vi "Example SM.vi"() -> ()   [LabVIEW 2020]
uses:
  FINS/FINS_header.ctl
  FINS/FINS CMD.ctl
  subvi/task.ctl
  FINS/FINS TCP.lvlib
panel:
  out "Waveform Chart 2":u32(graph)
  out "x-y 2":u32
  out "Array":sgl[](array[numeric])
  out "x-y":u32
  in  "address":u16=146
  out "Waveform Chart":sgl[][](graph)
  in  "stop":bool
  out "error o":errorcluster
  out "Numeric":sgl format="%.1f"
  out "data":bool[][](array[boolean])
  out "data":u8[](array[numeric])
  out "RSP":bool
  out "server Header":T1={"resp req"=FALSE, "cmd resp"=FALSE, "SID"=255, "DNA"=2, "DA1"=2, "DA2"=2, "SA1"=0, "SA2"=255, "SNA"=255} {"SNA" max=127 format="%x"; "SA2" max=254 step=1 format="%x"; "SA1" format="%x"; "DA2" max=254 step=1 format="%x"; "DA1" format="%x"; "DNA" max=127 step=1 format="%x"}
  out "server CMD":T2
  out "FINS Header":T1 {"SNA" max=127 format="%x"; "SA2" max=254 step=1 format="%x"; "SA1" format="%x"; "DA2" max=254 step=1 format="%x"; "DA1" format="%x"; "DNA" max=127 step=1 format="%x"}
  in  "SA1":u8 format="%x"
  out "Client Node":u32=10 format="%x"
  out "Server Node":u32=10 format="%x"
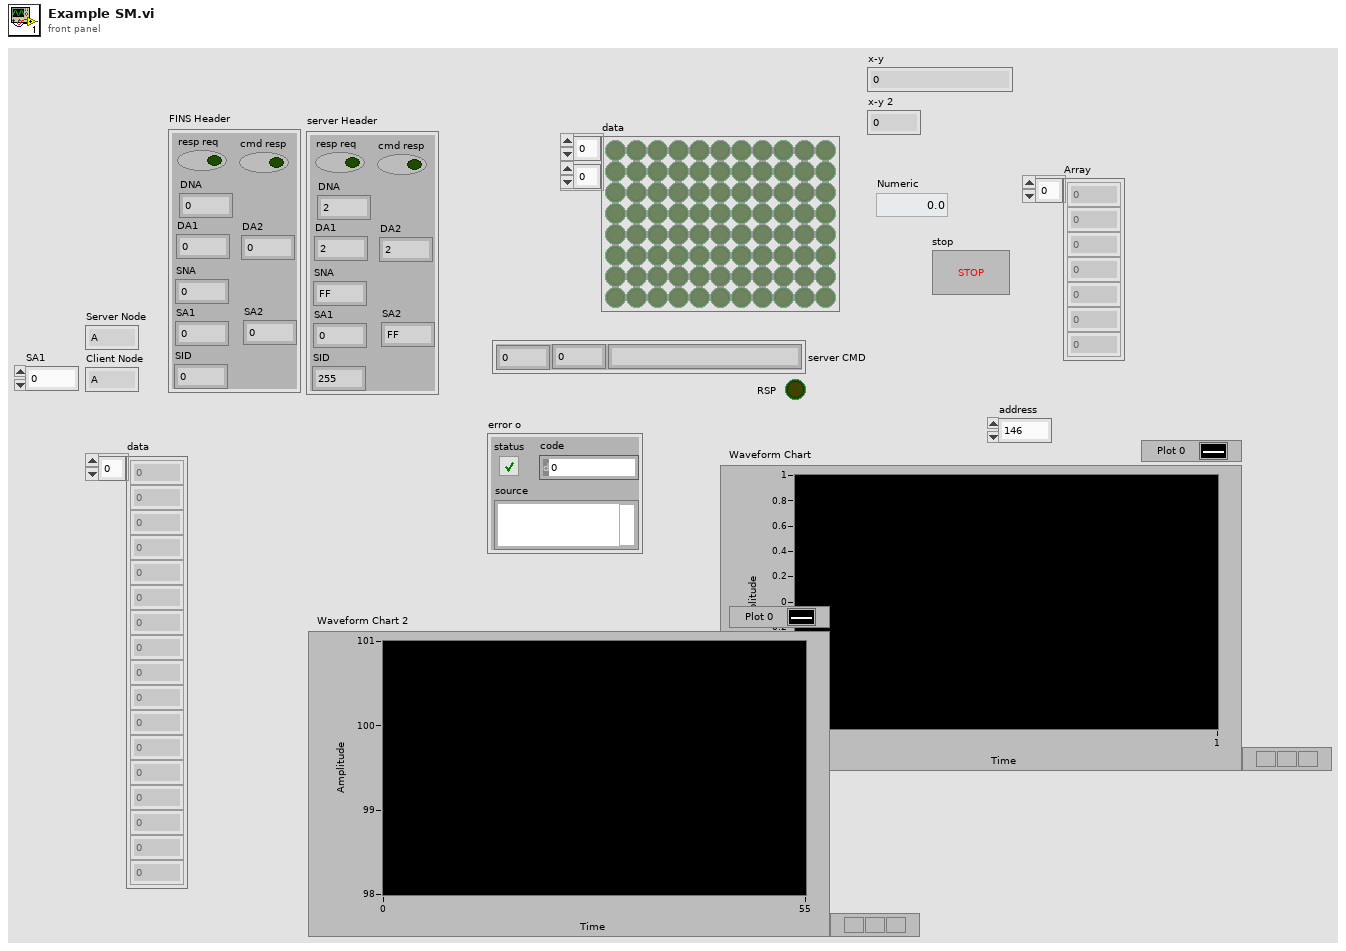
[diagram p1: front panel]
types:
  T1 = typedef "FINS TCP.lvlib/FINS_header.ctl" = cluster{"resp req":bool, "cmd resp":bool, "SID":u8, "DNA":u8, "DA1":u8, "DA2":u8, "SA1":u8, "SA2":u8, "SNA":u8}
  T2 = typedef "FINS TCP.lvlib/FINS CMD.ctl" = cluster{"MR":u8, "SR":u8, "name":string}
  T3 = typedef "task.ctl" = enum16{"connect", "send", "send-recv", "receive", "disconnect"}
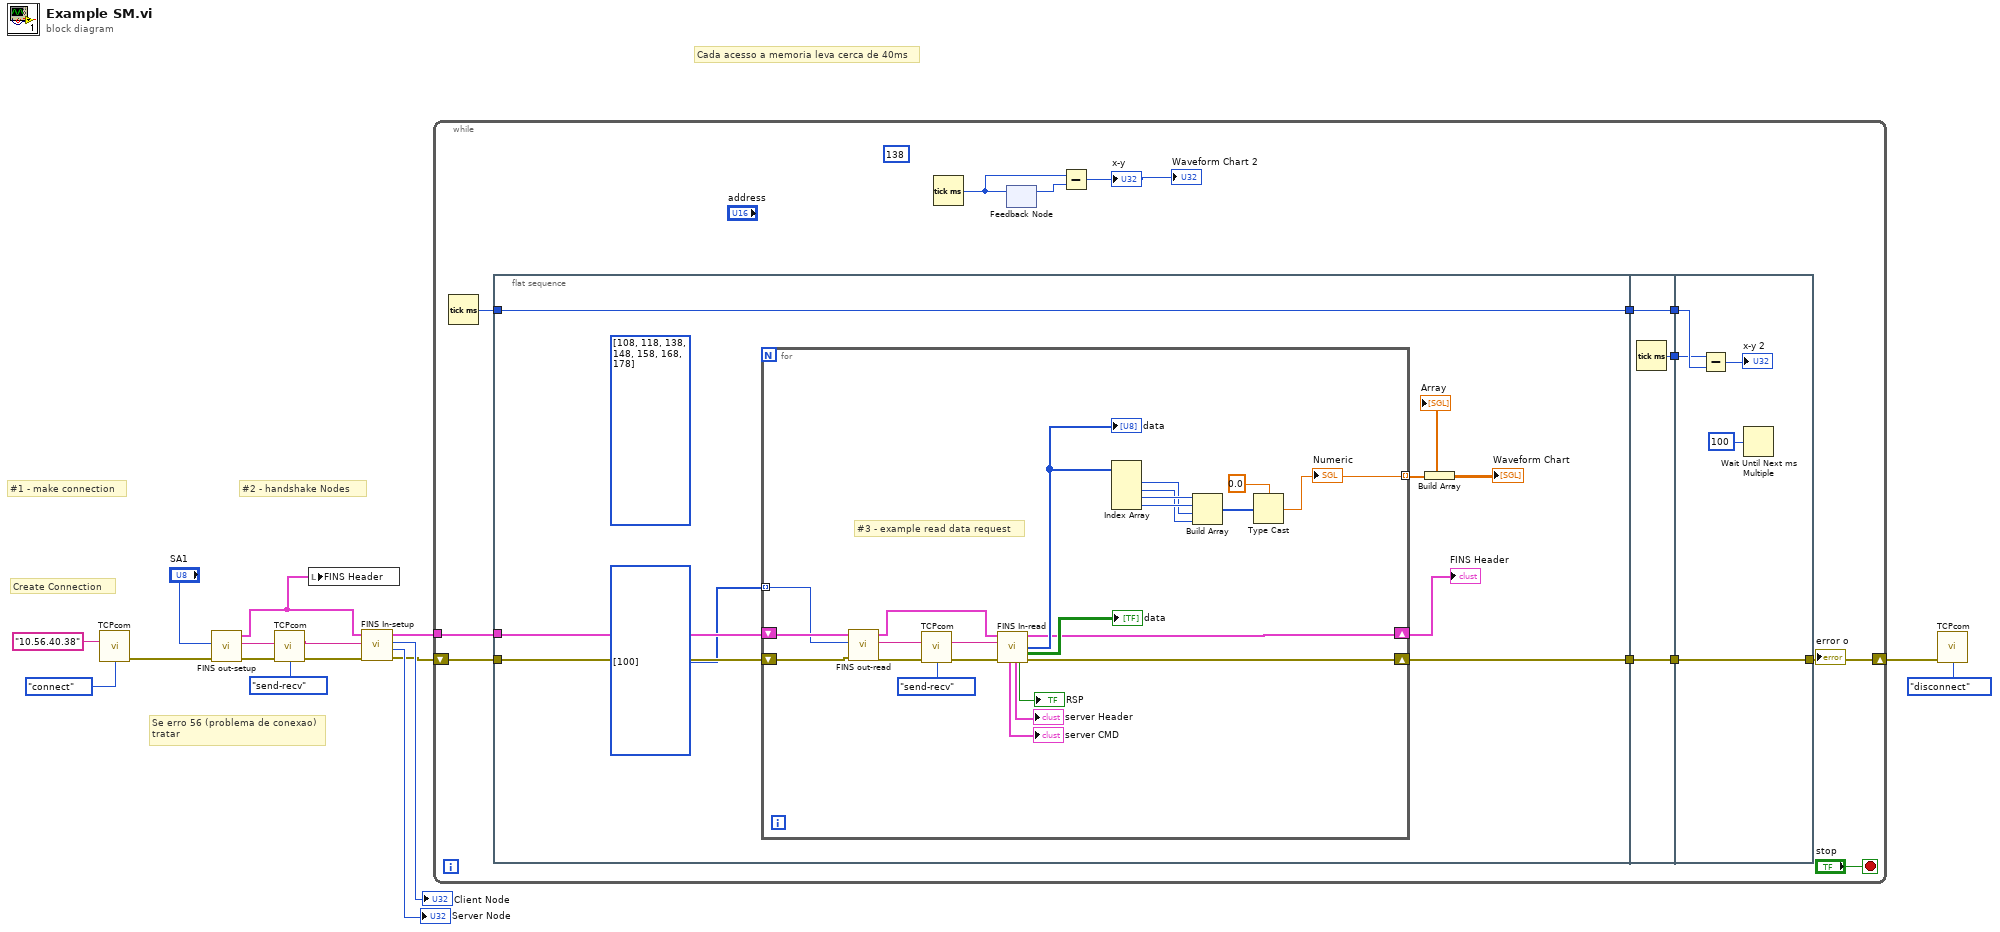
[diagram p0: block diagram]
diagram:
  # "Cada acesso a memoria leva cerca de 40ms"
  # "Se erro 56 (problema de conexao)\ntratar"
  # "#2 - handshake Nodes"
  # "#1 - make connection"
  # "Create Connection"
  n1 = call "TCPcom.vi"("string"="10.56.40.38" ("address"), "task"=task."connect") -> ("error out"=w15:errorcluster)  [unwired: 12 in, 1 out]
  n2 = call "FINS out-setup.vi"("error i"=w15, "SA1"="SA1") -> ("error o"=w13:errorcluster, "msg"=w14:string, "FINS Header"=w3:T1)  [unwired: 7 in]
  n3 = call "TCPcom.vi"("string"=w14, "error in"=w13, "task"=task."send-recv") -> ("data out"=w11:string, "error out"=w10:errorcluster)  [unwired: 11 in]
  n4 = local write "FINS Header"(w3) -> ()
  n5 = call "FINS In-setup.vi"("error i"=w10, "msg 3"=w11, "FINS Header i"=w3) -> ("error o"=w4:errorcluster, "Server Node"=→"Server Node":u32, "Client Node"=→"Client Node":u32, "FINS Header o"=w5:T1)  [unwired: 5 in]
  n6 = while {
    tunnel: w5 -> [w29]
    shift-right: [w27] -> w1
    shift-left: w4 -> [w28]
    stop <- "stop" stop-if-true
    (unwired) u16 138 ("address")
    n7 = Tick Count (ms)() -> (millisecond timer value=w23:u32)
    n8 = flat-sequence {
      tunnel: w29 -> [w37]
      tunnel: w28 -> [w36]
      tunnel: [w35] -> w22
      tunnel: [w30] -> w20
      tunnel: w23 -> [w30]
      tunnel: w22 -> [w63]
      tunnel: [w63] -> w21
      tunnel: w20 -> [w62]
      tunnel: [w62] -> w19
      tunnel: [w61] -> w18
      tunnel: [w68] -> w27
      tunnel: w21 -> [w68]
      tunnel: w19 -> [w66]
      tunnel: w18 -> [w65]
      frame #0 {
        (unwired) u16[] [108, 118, 138, 148, 158, 168, 178]
        n9 = for {
          shift-right: [w50] -> w35
          shift-left: w36 -> [w58]
          tunnel: u16[] [100] -> [w40] mode=indexing
          tunnel: [w39] -> w33 mode=indexing
          shift-right: [w38] -> w31
          shift-left: w37 -> [w59]
          # "#3 - example read data request"
          n10 = call "FINS out-read.vi"("error i"=w58, "address"=w40, "FINS Header 2"=w59) -> ("error o"=w56:errorcluster, "msg"=w57:string, "FINS Header"=w49:T1)  [unwired: 6 in]
          n11 = call "TCPcom.vi"("string"=w57, "error in"=w56, "task"=task."send-recv") -> ("data out"=w55:string, "error out"=w54:errorcluster)  [unwired: 11 in]
          n12 = call "FINS In-read.vi"("FINS Header i"=w49, "msg 3"=w55, "error i"=w54) -> ("FINS Header o"=w38:T1, 8:"data"=w41:u8[], 10:"data"=→"data":bool[][], "CMD"=→"server CMD":T2, "FINS Header 2"=→"server Header":T1, "RSP"=→"RSP":bool, "error o"=w50:errorcluster)  [unwired: 6 in]
          "data" <- w41
          n13 = Index Array(array=w41) -> (element #1=w44:u8, element #2=w43:u8, element #3=w46:u8, element #4=w45:u8)  [unwired: 4 in]
          n14 = Build Array(w46, w45, w44, w43) -> (w42:u8[])
          n15 = Type Cast(type=sgl 0.0 ("Numeric"), x=w42) -> (*(type *) &x=w39:sgl)
          "Numeric" <- w39
        }
        "Array" <- w33
        "FINS Header" <- w31
        n16 = Build Array(w33) -> (→"Waveform Chart":sgl[][])
      }
      frame #1 {
        n17 = Tick Count (ms)() -> (millisecond timer value=w61:u32)
      }
      frame #2 {
        n18 = Subtract(x=w65, y=w66) -> (x-y=→"x-y 2":u32)
        n19 = Wait Until Next ms Multiple(millisecond multiple=u32 100) -> ()  [unwired: 1 out]
      }
    }
    n20 = Tick Count (ms)() -> (millisecond timer value=w24:u32)
    n21 = feedback-in #1(w24) -> ()
    n22 = feedback #1() -> (w25:u32)  [unwired: 1 in]
    n23 = Subtract(x=w24, y=w25) -> (x-y=→"x-y" →"Waveform Chart 2":u32)
    "error o" <- w27
  }
  n24 = call "TCPcom.vi"("error in"=w1, "task"=task."disconnect") -> ()  [unwired: 12 in, 2 out]
